vi "dfd_FXP Simu.vi"(5 "input range":dbl=1.0, 6 "input selector":enum16{"FXP", "Integer", "Double"}(ring), 7 "init? (T)":bool=TRUE, 8 "error in (no error)":errorcluster, 9 "filtering statistics in":T3(array[cluster]) {"statistics information"."min value" format="%.2f"; "statistics information"."max value" format="%.2f"; "Quantizer Source" items=["Coefficients a/k"=0, "Coefficients b/v"=7, "Input"=1, "Output"=2, "Multiplicand"=3, "Product"=4, "Sum"=5, "Delay"=6]}, 10 "filter":T4 {"mSRate_QSettings"."source" items=["Coef a/k"=0, "Coef b/v"=7, "Input"=1, "Output"=2, "Multiplicand"=3, "Product"=4, "Sum"=5, "Delay"=6, "Gain"=8]}, 11 "signal in":dbl[](array[numeric])) -> (0 "error out":errorcluster, 1 "filtering statistics out":T3(array[cluster]) {"statistics information"."min value" format="%.2f"; "statistics information"."max value" format="%.2f"; "Quantizer Source" items=["Coefficients a/k"=0, "Coefficients b/v"=7, "Input"=1, "Output"=2, "Multiplicand"=3, "Product"=4, "Sum"=5, "Delay"=6]}, 2 "integer signal out":i32[](array[numeric]), 3 "DBL signal out":dbl[](array[numeric]))   [LabVIEW 2017, in "NI_DigFilter_FXP.lvlib"]
uses:
  <vilib>/addons/Digital Filter Design/NI_DigFilter_FXP.lvlib
  <vilib>/addons/Digital Filter Design/_Objects.llb/DFD Filter Obj.ctl
  <vilib>/addons/Digital Filter Design/_Objects.llb/DFD Filter Coef.ctl
  <vilib>/addons/Digital Filter Design/_Objects.llb/DFD Filter Structure Type Selector.ctl
  <vilib>/addons/Digital Filter Design/_Objects.llb/dfd_Internal Quantization Settings.ctl
  <vilib>/addons/Digital Filter Design/_Objects.llb/dfd_Internal Quantization Srcs.ctl
  <vilib>/addons/Digital Filter Design/_Objects.llb/DFD Coef Norm Type.ctl
  <vilib>/addons/Digital Filter Design/_Objects.llb/DFD Quantization Sources.ctl
  <vilib>/addons/Digital Filter Design/_Objects.llb/DFD FXP Statistics Data.ctl
  <vilib>/addons/Digital Filter Design/FXPLib.llb/DFD FXP to I32 (vector).vi
  <vilib>/addons/Digital Filter Design/NI_DigFilterLicensed.lvlib
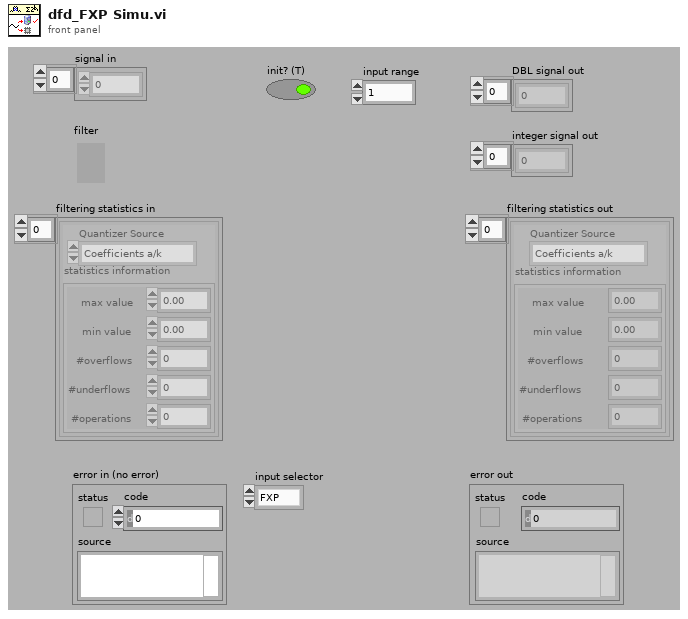
[diagram p1: front panel]
types:
  T1 = typedef "NI_DigFilterLicensed.lvlib/DFD Quantization Sources.ctl" = u16
  T2 = typedef "NI_DigFilterLicensed.lvlib/DFD FXP Statistics Data.ctl" = cluster{"max value":ext, "min value":ext, "#overflows":i32, "#underflows":i32, "#operations":i32}
  T3 = cluster{"Quantizer Source":T1, "statistics information":T2}[]
  T4 = typedef "NI_DigFilterLicensed.lvlib/DFD Filter Obj.ctl" = cluster{"mSRate_Fs":dbl, "mSRate_Version":string, "mSRate_Comments":string, "mSRate_OrgCoef":T5, "mSRate_CurCoef":T5, "mSRate_Quantized?":bool, "mSRate_QCoef":T5, "mSRate_QSettings":T7[], "mSRate_Order":i32, "mSRate_Scaling":cluster{"mSRate_ScaleByPowerOf2?":bool, "mSRate_ScaleType":T9}}
  T5 = typedef "NI_DigFilterLicensed.lvlib/DFD Filter Coef.ctl" = cluster{"type":T6, "gain":dbl, "coef a (k)":dbl[], "coef b (v)":dbl[]}
  T6 = typedef "NI_DigFilterLicensed.lvlib/DFD Filter Structure Type Selector.ctl" = enum16{"Undefined", "FIR Direct Form", "FIR Direct Form Transposed", "FIR Symmetric", "FIR Antisymmetric", "IIR Direct Form I", "IIR Direct Form I Transposed", "IIR Direct Form II", "IIR Direct Form II Transposed", "IIR Cascaded Second Order Sections Form I", "IIR Cascaded Second Order Sections Form I Transposed", "IIR Cascaded Second Order Sections Form II", "IIR Cascaded Second Order Sections Form II Transposed", "Lattice Allpass (basic sections)", "Lattice Allpass (one multiplier sections)", "Lattice Allpass (normalized sections)", "Lattice AR (basic sections)", "Lattice AR (one multiplier sections)", "Lattice AR (normalized sections)", "Lattice MA (minimum phase)", "Lattice MA (maximum phase)", "Lattice ARMA (basic sections)", "Lattice ARMA (one multiplier sections)", "Lattice ARMA (normalized sections)"}
  T7 = typedef "NI_DigFilterLicensed.lvlib/dfd_Internal Quantization Settings.ctl" = cluster{"source":T8, "wl":i16, "iwl":i16, "overflow mode":enum16{"Saturation", "Wrap"}, "rounding mode":enum16{"Nearest", "Truncation"}, "signed?":bool}
  T8 = typedef "NI_DigFilterLicensed.lvlib/dfd_Internal Quantization Srcs.ctl" = u16
  T9 = typedef "NI_DigFilterLicensed.lvlib/DFD Coef Norm Type.ctl" = enum16{"No Norm", "Time Domain 1-Norm", "Time Domain 2-Norm", "Time Domain Inf-Norm"}
  T10 = typedef "dfd_DFXP Operation Parameter.ctl" = cluster{"source":T8, "is floating?":bool, "o-mode":enum16{"Saturation", "Wrap"}, "q-mode":enum16{"Nearest", "Truncation"}, "wl":i16, "high limit":i64, "low limit":i64, "iwl":i16, "sign?":bool}
  T11 = typedef "dfd_DFXP Data Type (vector).ctl" = cluster{"Values":i64[], "wl":i16, "iwl":i16}
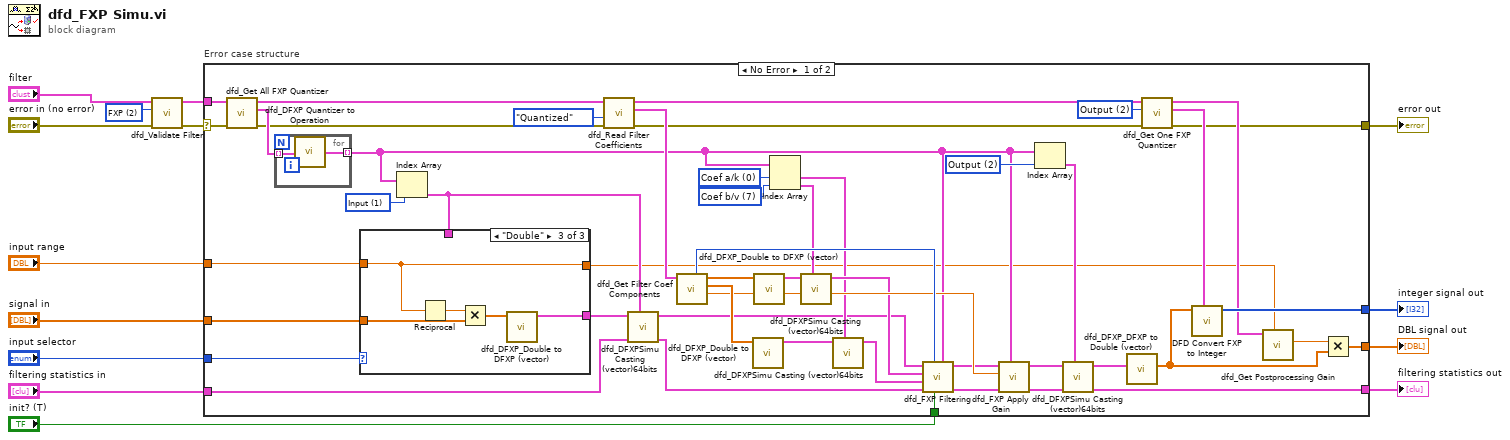
[diagram p0: block diagram]
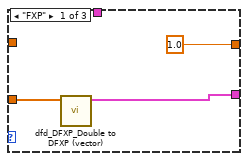
[diagram p2: hidden frame]
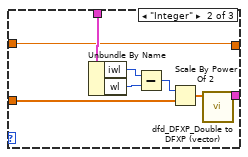
[diagram p3: hidden frame]
diagram:
  w9 = u16 2 items=["Auto", "FLP Only", "FXP"] ("check option")
  n1 = call <vilib>:"dfd_Validate Filter.vi"("error in (no error)"="error in (no error)", "check option"=w9, "filter in"="filter") -> ("error out"=w3:errorcluster, "filter out"=w4:T4)  [unwired: 7 out]
  n2 = case "Error case structure" shown="No Error" w3 {
    selector: w3 -> [w20 w82]
    tunnel: "filtering statistics in" -> [w23 _]
    tunnel: [w58 _] -> w13
    tunnel: "init? (T)" -> [w57 _]
    tunnel: [w56 _] -> w11
    tunnel: "signal in" -> [w27 _]
    tunnel: [w29 _] -> w10
    tunnel: w4 -> [w50 _]
    tunnel: "input range" -> [w28 _]
    tunnel: "input selector" -> [w26 _]
    tunnel: [w17 w82] -> w1
    frame No Error {
      w34 = T8 7 items=["Coef a/k"=0, "Coef b/v"=7, "Input"=1, "Output"=2, "Multiplicand"=3, "Product"=4, "Sum"=5, "Delay"=6, "Gain"=8] ("source")
      w36 = T8 0 items=["Coef a/k"=0, "Coef b/v"=7, "Input"=1, "Output"=2, "Multiplicand"=3, "Product"=4, "Sum"=5, "Delay"=6, "Gain"=8] ("source")
      w44 = T8 2 items=["Coef a/k"=0, "Coef b/v"=7, "Input"=1, "Output"=2, "Multiplicand"=3, "Product"=4, "Sum"=5, "Delay"=6, "Gain"=8] ("quantization source")
      w49 = T8 1 items=["Coef a/k"=0, "Coef b/v"=7, "Input"=1, "Output"=2, "Multiplicand"=3, "Product"=4, "Sum"=5, "Delay"=6, "Gain"=8] ("source")
      w46 = T8 2 items=["Coef a/k"=0, "Coef b/v"=7, "Input"=1, "Output"=2, "Multiplicand"=3, "Product"=4, "Sum"=5, "Delay"=6, "Gain"=8] ("quantization source")
      n3 = call <vilib>:"dfd_Get All FXP Quantizer.vi"("error in (no error)"=w20, "filter in"=w50) -> ("error out"=w19:errorcluster, "quantization settings"=w43:T7[], "filter out"=w48:T4)  [unwired: 7 out]
      n4 = for {
        tunnel: w43 -> [w81] mode=indexing
        tunnel: [w80] -> w35 mode=indexing
        n5 = call <vilib>:"dfd_DFXP Quantizer to Operation.vi"("quantizer"=w81) -> ("op params"=w80:T10)
      }
      n6 = Index Array(array=w35, index=w49) -> (element=w24:T10)
      n7 = case shown="\"Double\"" w26 {
        tunnel: w24 -> [_ w70 _]
        tunnel: w28 -> [_ w67 w75]
        tunnel: w27 -> [w66 w68 w77]
        tunnel: [w65 w69 w76] -> w25
        tunnel: [1.0 ("input range") w67 w75] -> w15
        frame "FXP" {
          n8 = call <vilib>:"dfd_DFXP_Double to DFXP (vector).vi"("value in"=w66) -> ("value out"=w65:T11)  [unwired: 10 out]
        }
        frame "Integer" {
          n9 = Unbundle By Name(w70) -> ("iwl"=w71:i16, "wl"=w72:i16)
          n10 = Subtract(x=w71, y=w72) -> (x-y=w73:i16)
          n11 = Scale By Power Of 2(n=w73, x=w68) -> (x*2^n=w74:dbl[])
          n12 = call <vilib>:"dfd_DFXP_Double to DFXP (vector).vi"("value in"=w74) -> ("value out"=w69:T11)  [unwired: 10 out]
        }
        frame "Double" {
          n13 = Reciprocal(x=w75) -> (1/x=w78:dbl)
          n14 = Multiply(x=w78, y=w77) -> (x*y=w79:dbl[])
          n15 = call <vilib>:"dfd_DFXP_Double to DFXP (vector).vi"("value in"=w79) -> ("value out"=w76:T11)  [unwired: 10 out]
        }
      }
      n16 = call <vilib>:"dfd_Read Filter Coefficients.vi"("error in (no error)"=w19, "coef source"=enum16{"Original", "Current", "Quantized"}."Quantized", "filter in"=w48) -> ("error out"=w18:errorcluster, "filter coef"=w62:T5, "filter out"=w42:T4)  [unwired: 6 out]
      n17 = call <vilib>:"dfd_DFXPSimu Casting (vector)64bits.vi"("op params"=w24, "filtering statistics in"=w23, "Value in"=w25) -> ("filtering statistics out"=w22:T3, "Value out"=w21:T11)  [unwired: 1 in, 6 out]
      n18 = call <vilib>:"dfd_Get Filter Coef Components.vi"("filter coef"=w62) -> ("gain"=w53:dbl, "coef a (k)"=w54:dbl[], "coef b (v)"=w55:dbl[], "type"=w63:T6)  [unwired: 1 in, 6 out]
      n19 = call <vilib>:"dfd_DFXP_Double to DFXP (vector).vi"("value in"=w54) -> ("value out"=w38:T11)  [unwired: 10 out]
      n20 = call <vilib>:"dfd_DFXP_Double to DFXP (vector).vi"("value in"=w55) -> ("value out"=w40:T11)  [unwired: 10 out]
      n21 = Index Array(array=w35, index #1=w36, index #2=w34) -> (element #1=w33:T10, element #2=w32:T10)
      n22 = call <vilib>:"dfd_DFXPSimu Casting (vector)64bits.vi"("op params"=w32, "Value in"=w40) -> ("Value out"=w39:T11)  [unwired: 2 in, 7 out]
      n23 = call <vilib>:"dfd_DFXPSimu Casting (vector)64bits.vi"("op params"=w33, "Value in"=w38) -> ("Value out"=w37:T11)  [unwired: 2 in, 7 out]
      n24 = call <vilib>:"dfd_FXP Filtering.vi"("FXPOPs"=w35, "init? (T)"=w57, "struct typ"=w63, "filtering statistics in"=w22, "coef a"=w37, "coef b"=w39, "X"=w21) -> ("filtering statistics out"=w60:T3, "filtered X"=w47:T11)  [unwired: 3 out]
      n25 = call <vilib>:"dfd_FXP Apply Gain.vi"("FXPOPs"=w35, "filtering statistics in"=w60, "gain"=w53, "before-gain X"=w47) -> ("filtering statistics out"=w59:T3, "after-gain X"=w52:T11)  [unwired: 6 out]
      n26 = Index Array(array=w35, index=w46) -> (element=w45:T10)
      n27 = call <vilib>:"dfd_DFXPSimu Casting (vector)64bits.vi"("op params"=w45, "filtering statistics in"=w59, "Value in"=w52) -> ("filtering statistics out"=w58:T3, "Value out"=w51:T11)  [unwired: 1 in, 6 out]
      n28 = call <vilib>:"dfd_DFXP_DFXP to Double (vector).vi"("Value in"=w51) -> ("DBL"=w30:dbl[])  [unwired: 10 out]
      n29 = call <vilib>:"dfd_Get One FXP Quantizer.vi"("error in (no error)"=w18, "quantization source"=w44, "filter in"=w42) -> ("error out"=w17:errorcluster, "quantization settings"=w41:T7, "filter out"=w31:T4)  [unwired: 6 out]
      n30 = call-poly <vilib>:"DFD Convert FXP to Integer.vi"("quantization settings"=w41, "FXP values"=w30) -> ("I32 values"=w56:i32[])  [unwired: 1 in, 8 out]
      n31 = call <vilib>:"dfd_Get Postprocessing Gain.vi"("input range"=w15, "filter"=w31) -> ("DBL gain"=w16:dbl)  [unwired: 9 out]
      n32 = Multiply(x=w16, y=w30) -> (x*y=w29:dbl[])
    }
    frame Error {
    }
  }
  "filtering statistics out" <- w13
  "error out" <- w1
  "DBL signal out" <- w10
  "integer signal out" <- w11
